vi "Initialize.vi"(8 "error in (no error)":errorcluster, 11 "ChromaAcLoad in":refnum<class "ChromaAcLoad.lvclass">) -> (0 "error out":errorcluster, 3 "ChromaAcLoad out":refnum<class "ChromaAcLoad.lvclass">)   [LabVIEW 2018, in "AcPwrPlugins.lvlib" / "ChromaAcLoad.lvclass"]
doc: "This VI estabilishes communication ot the instrument and optionally sets the initial state of the following session attributes:\n\n C63800_ATTR_RANGE_CHECK \n C63800_ATTR_QUERY_INSTR_STATUS \n C63800_ATTR_CACHE \n C63800_ATTR_SIMULATE \n C63800_ATTR_RECORD_COERCIONS \n\n- Opens a session to the specified device using the interface and address you specify for the Resource Name parameter.\n\n- If the ID Query parameter is set to VI_TRUE, this function queries the instrument ID and checks that it is valid for this instrument driver.\n\n- If the Reset parameter is set to VI_TRUE, this function resets the instrument to a known state.\n\n- Sends initialization commands to set the instrument to the state necessary for the operation of the instrument driver.\n\n- Returns a ViSession handle that you use to identify the instrument in all subsequent instrument driver function calls.\n\nNote: This function creates a new session each time you invoke it. Although you can open more than one IVI session for the same resource, it is best not to do so. You can use the same session in multiple program threads. You can use the C63800_LockSession and C63800_UnlockSession functions to protect sections of code that require exclusive access to the resource."
uses:
  ChromaAcLoad.lvclass
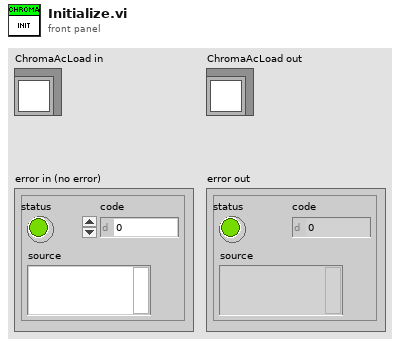
[diagram p1: front panel]
types:
  T1 = cluster{"f":bool, "Instrument Handle out 2":refnum<k15>}[]
  T2 = typedef "AcPwrPlugins.lvlib/ChromaAcLoad.lvclass/Device(s)Settings.ctl" = cluster{"Configuration Mode":enum16{"Constant Voltage (DC)", "Constant Power (DC)", "Constant Power (AC)", "Constant Current (DC)", "Constant Current (AC)", "Constant Resistance (DC)", "Constant Resistance (AC)", "Rectified Mode (DC)", "Inrush (AC)", "RLC CP (AC)", "RLC (AC)"}, "Phases":cluster{"Handle":string, "Name":string, "Phase Select":i32, "Instrument Options":string, "id query (T)":bool, "reset device (T)":bool, "Load Short Circuited":bool, "Line Synchronization":bool, "Load Current (A/Arms)":dbl, "Load Voltage (V/Vrms)":dbl, "Load Power (W)":dbl, "Load Resistance (Ohms)":dbl, "Load Current Peak Limit (A)":dbl, "Load Current Limit (A/Arms)":dbl, "Load Power Limit (W)":dbl, "Synch Frequency (Hz)":dbl, "Priority":enum16{"CF Only", "PF Only", "Both (CF)", "Both (PF)"}, "Crest Factor":dbl, "Power Factor":dbl, "Slew Rate":cluster{"Rise Slew Rate (A/ms)":i32, "Fall Slew Rate (A/ms)":i32}, "LC/RLC Mode":cluster{"Capacitance (uF)":i32, "Inductance (uH)":i32, "Series Resistance (Ohm)":dbl, "Parallel Resistance (Ohm)":dbl}, "Timing":cluster{"TimingOn":enum16{""}, "Hours":u32, "Minutes":u32, "Seconds":dbl, "CutoffVoltage":dbl}, "Connected":bool}[], "MeasName":string}
  T3 = typedef "AcPwrPlugins.lvlib/ChromaAcLoad.lvclass/Measurements.ctl" = cluster{"Handle":string, "Name":string, "Enabled":bool, "Measurement Value":dbl, "Hold Peak Current Measurement":bool, "btnMeasFetch":bool, "ProtectionStatusString":string, "Measurement Type":T4}[]
  T4 = typedef "AcPwrPlugins.lvlib/ChromaAcLoad.lvclass/MeasurementType.ctl" = enum16{"Voltage (Vrms or V)", "Current (Arms or A)", "Power (W)", "Peak Voltage (V)", "Peak Current (A)", "Peak Power (W)", "Frequency (Hz)", "Resistance (Ohms)", "Voltage Overshoot (V)", "Positive Peak Current (A)", "Voltage Undershoot (V)", "Negative Peak Current (A)", "Apparent Power (VA)", "Reacitive Power (VAR)", "Voltage THD", "Power Factor", "Current's Crest Factor"}
  T5 = cluster{"Handle":string, "Name":string, "Phase Select":i32, "Instrument Options":string, "id query (T)":bool, "reset device (T)":bool, "Load Short Circuited":bool, "Line Synchronization":bool, "Load Current (A/Arms)":dbl, "Load Voltage (V/Vrms)":dbl, "Load Power (W)":dbl, "Load Resistance (Ohms)":dbl, "Load Current Peak Limit (A)":dbl, "Load Current Limit (A/Arms)":dbl, "Load Power Limit (W)":dbl, "Synch Frequency (Hz)":dbl, "Priority":enum16{"CF Only", "PF Only", "Both (CF)", "Both (PF)"}, "Crest Factor":dbl, "Power Factor":dbl, "Slew Rate":cluster{"Rise Slew Rate (A/ms)":i32, "Fall Slew Rate (A/ms)":i32}, "LC/RLC Mode":cluster{"Capacitance (uF)":i32, "Inductance (uH)":i32, "Series Resistance (Ohm)":dbl, "Parallel Resistance (Ohm)":dbl}, "Timing":cluster{"TimingOn":enum16{""}, "Hours":u32, "Minutes":u32, "Seconds":dbl, "CutoffVoltage":dbl}, "Connected":bool}[]
  T6 = cluster{"Handle Connected?":bool, "Instrument Handle":refnum<k15>}
  T7 = cluster{"Handle Connected?":bool, "Instrument Handle":refnum<k15>}[]
  T8 = cluster{"Handle":string, "Name":string, "Phase Select":i32, "Instrument Options":string, "id query (T)":bool, "reset device (T)":bool, "Load Short Circuited":bool, "Line Synchronization":bool, "Load Current (A/Arms)":dbl, "Load Voltage (V/Vrms)":dbl, "Load Power (W)":dbl, "Load Resistance (Ohms)":dbl, "Load Current Peak Limit (A)":dbl, "Load Current Limit (A/Arms)":dbl, "Load Power Limit (W)":dbl, "Synch Frequency (Hz)":dbl, "Priority":enum16{"CF Only", "PF Only", "Both (CF)", "Both (PF)"}, "Crest Factor":dbl, "Power Factor":dbl, "Slew Rate":cluster{"Rise Slew Rate (A/ms)":i32, "Fall Slew Rate (A/ms)":i32}, "LC/RLC Mode":cluster{"Capacitance (uF)":i32, "Inductance (uH)":i32, "Series Resistance (Ohm)":dbl, "Parallel Resistance (Ohm)":dbl}, "Timing":cluster{"TimingOn":enum16{""}, "Hours":u32, "Minutes":u32, "Seconds":dbl, "CutoffVoltage":dbl}, "Connected":bool}
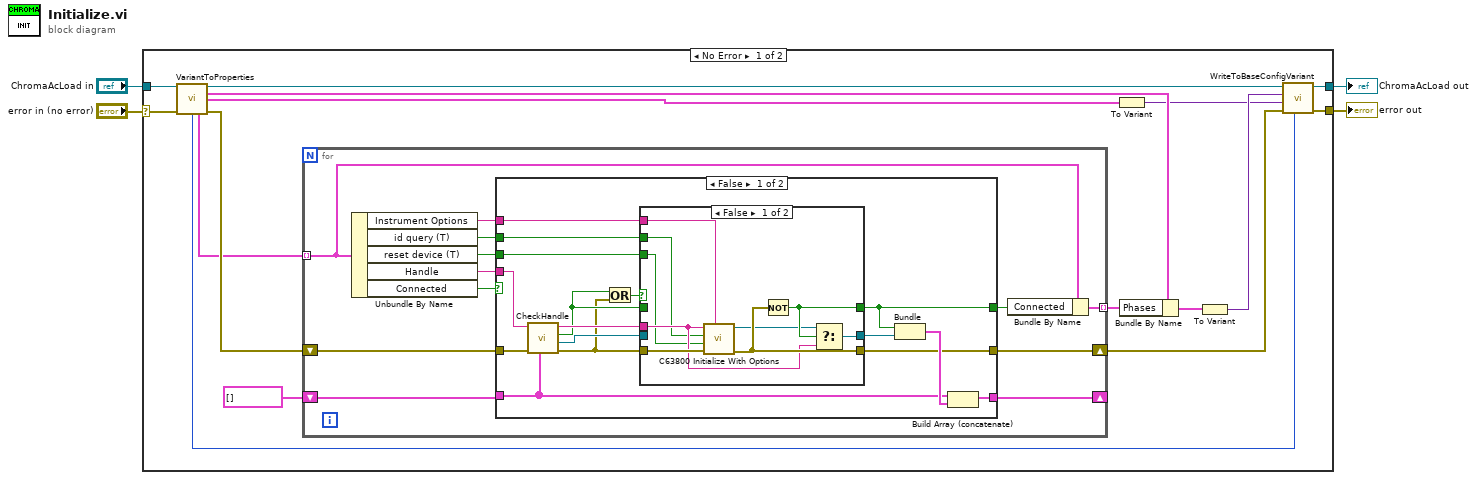
[diagram p0: block diagram]
diagram:
  n1 = case shown="No Error" "error in (no error)" {
    selector: "error in (no error)" -> [w19 w65]
    tunnel: "ChromaAcLoad in" -> [w20 w64]
    tunnel: [w13 w64] -> w2
    tunnel: [w12 w65] -> w1
    frame No Error {
      n2 = call "VariantToProperties.vi"("ChromaAcLoad"=w20, "error in (no error)"=w19) -> ("ChromaAcLoad"=w10:refnum<class "ChromaAcLoad.lvclass">, "Device Properties"=w9:T2, "Meas"=w6:T3, "Measurement Refresh Time (ms)"=w5:u32, "Phases"=w8:T5, "error out"=w17:errorcluster)  [unwired: 7 in, 1 out]
      n3 = for {
        shift-right: [w31] -> w11
        shift-left: w17 -> [w32]
        tunnel: w8 -> [w25] mode=indexing
        shift-right: [w29] -> _
        shift-left: T1 [] -> [w30]
        tunnel: [w24] -> w16 mode=indexing
        n4 = Unbundle By Name(w25) -> ("Instrument Options"=w23:string, "id query (T)"=w22:bool, "reset device (T)"=w21:bool, "Handle"=w28:string, "Connected"=w27:bool)
        n5 = case shown="False" w27 {
          selector: w27 -> [_ w63]
          tunnel: [w42 w63] -> w26
          tunnel: w28 -> [w48 _]
          tunnel: [w43 w62] -> w31
          tunnel: w32 -> [w36 w62]
          tunnel: w30 -> [w33 w61]
          tunnel: [w46 w61] -> w29
          tunnel: w23 -> [w41 _]
          tunnel: w22 -> [w40 _]
          tunnel: w21 -> [w39 _]
          frame False {
            n6 = call "CheckHandle.vi"("Array"=w33, "Error In"=w36, "Handle In"=w48) -> ("Error Out"=w34:errorcluster, "Instrument Handle"=w38:refnum<k15>, "Handle Connected?"=w35:bool, "Handle Out"=w37:string)  [unwired: 5 in]
            n7 = Or(x=w35, y=w34) -> (x .or. y?=w47:bool)
            n8 = case shown="False" w47 {
              tunnel: [w56 w59] -> w42
              tunnel: w37 -> [w53 _]
              tunnel: w34 -> [w54 w60]
              tunnel: [w55 w60] -> w43
              tunnel: w35 -> [_ w59]
              tunnel: [w57 w58] -> w45
              tunnel: w38 -> [_ w58]
              tunnel: w41 -> [w50 _]
              tunnel: w40 -> [w52 _]
              tunnel: w39 -> [w51 _]
              frame False {
                n9 = call <instrlib>:"C63800 Initialize With Options.vi"("Option String"=w50, "error in (no error)"=w54, "Reset Device"=w51, "ID Query"=w52, "Resource Name"=w53) -> ("error out"=w55:errorcluster, "Instrument Handle out"=w49:refnum<k15>)  [unwired: 5 in]
                n10 = Not(x=w55) -> (.not. x?=w56:bool)
                n11 = Select(t=w49, s=w56, f=w53) -> (s? t:f=w57:refnum<k15>)
              }
              frame True {
              }
            }
            n12 = Bundle("Handle Connected?"=w42, "Instrument Handle"=w45) -> (w44:T6)  [unwired: 1 in]
            n13 = Build Array (concatenate)(w33, w44) -> (w46:T7)
          }
          frame True {
          }
        }
        n14 = Bundle By Name(cluster=w25, "Connected"=w26) -> (w24:T8)
      }
      n15 = To Variant(anything=w6) -> (Variant=w7:variant)
      n16 = Bundle By Name(cluster=w9, "Phases"=w16) -> (w15:T2)
      n17 = To Variant(anything=w15) -> (Variant=w14:variant)
      n18 = call "WriteToBaseConfigVariant.vi"("Measurement Refresh Time (ms)"=w5, "error in (no error)"=w11, "Meas"=w7, "Config"=w14, "ChromaAcLoad in"=w10) -> ("error out"=w12:errorcluster, "ChromaAcLoad out"=w13:refnum<class "ChromaAcLoad.lvclass">)  [unwired: 5 in]
    }
    frame Error {
    }
  }
  "error out" <- w1
  "ChromaAcLoad out" <- w2
